vi "Config Dev Shunt.vi"(8 "error in":errorcluster, 11 "VISA resource name":refnum<visa-resource-name>) -> (0 "error out":errorcluster, 3 "VISA resource name out":refnum<visa-resource-name>)   [LabVIEW 2019, in "Andeen-Hagerling 2700(400 firmware).lvlib"]
doc: "Sets the span between the DBndLo and DBndUp in pF (or jpF)."
uses:
  <instrlib>/Andeen-Hagerling 2700(400 firmware)/Andeen-Hagerling 2700(400 firmware).lvlib
panel:
  in  "Shunt (auto)":enum16{"off", "on", "auto"}(ring)=enum."auto"
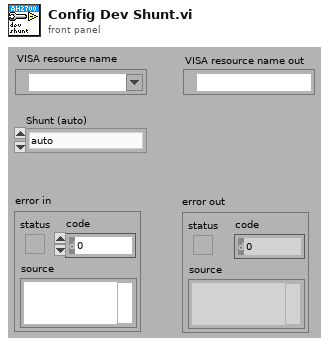
[diagram p1: front panel]
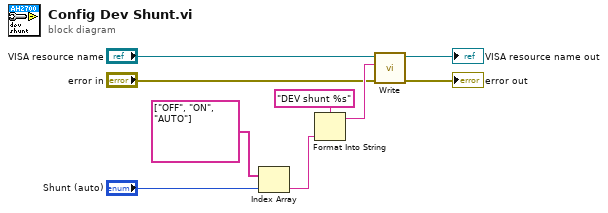
[diagram p0: block diagram]
diagram:
  n1 = Index Array(array=string[] ["OFF", "ON", "AUTO"], index="Shunt (auto)") -> (element=w1:string)
  n2 = Format Into String(format string="DEV shunt %s", w1) -> (resulting string=w8:string)  [unwired: 2 in, 1 out]
  n3 = call <instrlib>:"Write.vi"("error in"="error in", "command"=w8, "VISA resource name"="VISA resource name") -> ("error out"=→"error out":errorcluster, "VISA resource name out"=→"VISA resource name out":refnum<visa-resource-name>)  [unwired: 7 in]
